vi "Initialize UI Process.vi"(8 "error in (no error)":errorcluster, 10 "Consumer Queues in":T1, 11 "Test Stand.lvclass":refnum<class "Generic Test Stand.lvclass">) -> (0 "error out":errorcluster, 2 "Consumer Queues out":T1)   [LabVIEW 2019, in "TS Framework.lvlib"]
uses:
  TS Framework.lvlib
  Consumer Queues.ctl
  UI Process/Generic UI Command/Generic UI Process Command.lvclass
  DAC Process/Generic DAC Command/Generic DAC Process Command.lvclass
  Trig Process/Generic Trig Command/Generic Trig Process Command.lvclass
  Generic Test Stand/Generic Test Stand.lvclass
  UI Process/Init UI Process/Init UI Process.lvclass
  UI Process/Init UI Process/Init UI Process.lvclass/Init UI Process.ctl
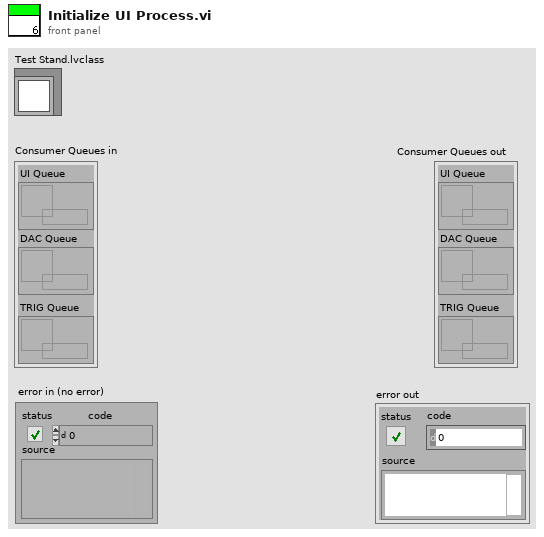
[diagram p1: front panel]
types:
  T1 = typedef "TS Framework.lvlib/Consumer Queues.ctl" = cluster{"UI Queue":refnum<queue>, "DAC Queue":refnum<queue>, "TRIG Queue":refnum<queue>}
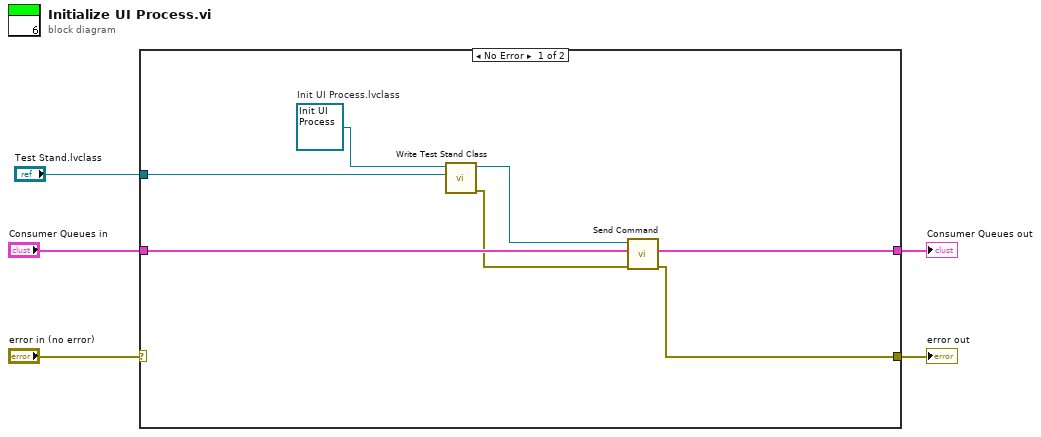
[diagram p0: block diagram]
diagram:
  n1 = case shown="No Error" "error in (no error)" {
    selector: "error in (no error)" -> [_ w14]
    tunnel: "Consumer Queues in" -> [w12 w13]
    tunnel: [w11 w13] -> w3
    tunnel: [w10 w14] -> w2
    tunnel: "Test Stand.lvclass" -> [w8 _]
    frame No Error {
      w9 = refnum<class "Init UI Process.lvclass"> refnum  # Init UI Process.lvclass
      n2 = call "Write Test Stand Class.vi"("Generic Test Stand.lvclass"=w8, "Init UI Process in"=w9) -> ("error out"=w6:errorcluster, "Init UI Process out"=w7:refnum<class "Init UI Process.lvclass">)  [unwired: 8 in]
      n3 = call-dynamic "Send Command.vi"("error in (no error)"=w6, "Consumer Queues in"=w12, "UI Process Command in"=w7) -> ("error out"=w10:errorcluster, "Consumer Queues out"=w11:T1)  [unwired: 7 in]
    }
    frame Error {
    }
  }
  "Consumer Queues out" <- w3
  "error out" <- w2
